vi "jsq_encode.vi"(8 "error in (no error)":errorcluster, 10 "Sequence":T1[](array[typedef])) -> (0 "error out":errorcluster, 2 "JSON string":string="[\r\n]")   [LabVIEW 2015, in "oskar_tools.lvlib"]
uses:
  oskar_tools.lvlib
  seq_line.ctl
  <vilib>/regexp/Match Regular Expression.xnode
  <vilib>/addons/_JKI.lib/Serialization/JSON/JKI JSON Serialization.lvlib
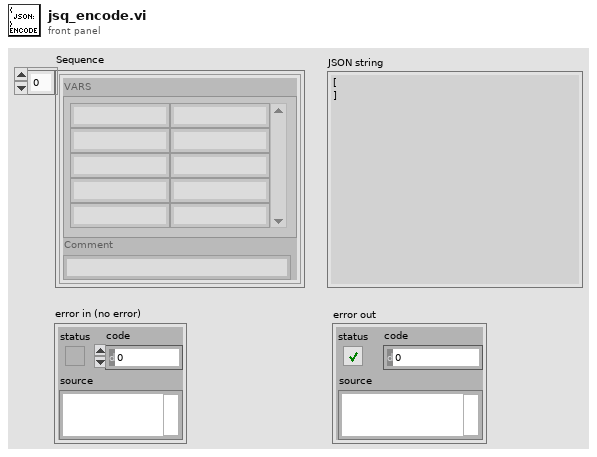
[diagram p1: front panel]
types:
  T1 = typedef "oskar_tools.lvlib/seq_line.ctl" = cluster{"VARS":string[][], "Comment":string}
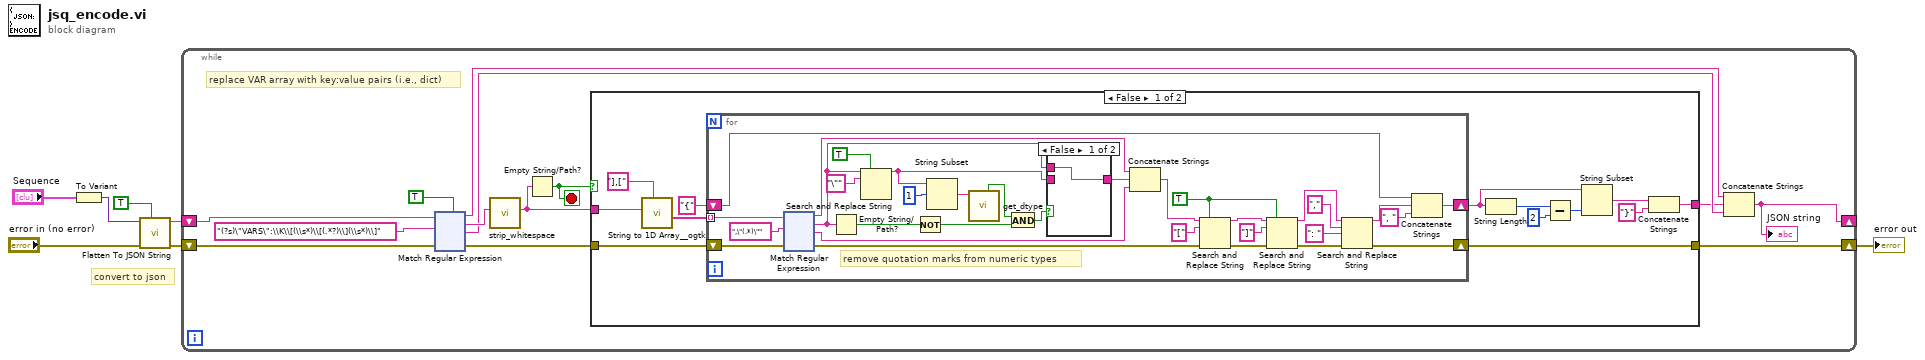
[diagram p0: block diagram]
diagram:
  # "convert to json"
  n1 = To Variant(anything="Sequence") -> (Variant=w7:variant)
  n2 = call <vilib>:"Flatten To JSON String.vi"("Multiline (T)"=TRUE, "error in (no error)"="error in (no error)", "Variant"=w7) -> ("error out"=w2:errorcluster, "JSON String"=w4:string)  [unwired: 7 in]
  n3 = while {
    shift-right: [w17] -> _
    shift-left: w4 -> [w19]
    shift-right: [w8] -> w1
    shift-left: w2 -> [w10]
    stop <- w15 stop-if-true
    # "replace VAR array with key:value pairs (i.e., dict)"
    n4 = xnode "Match Regular Expression"("input string"=w19, "regular expression"="(?s)\"VARS\":\\K\\[(\\s*)\\[(.*?)\\](\\s*)\\]", "error in"=w10, "multiline? (F)"=TRUE) -> ("before match"=w18:string, "whole match"=w14:string, "after match"=w12:string, "error out"=w9:errorcluster)  [unwired: 2 in, 1 out]
    n5 = call "strip_whitespace.vi"("String in"=w14) -> ("String out"=w13:string)  [unwired: 10 in]
    n6 = Empty String/Path?(string/path=w13) -> (empty?=w15:bool)
    n7 = case shown="False" w15 {
      tunnel: w13 -> [w33 w183]
      tunnel: [w28 w183] -> w11
      tunnel: w9 -> [w22 w182]
      tunnel: [w21 w182] -> w8
      frame False {
        n8 = call <userlib>:"String to 1D Array__ogtk.vi"("delimiter (Tab)"="],[" ("format string"), "string"=w33) -> ("Array of Strings"=w31:string[])  [unwired: 9 in]
        n9 = for {
          tunnel: w31 -> [w53] mode=indexing
          shift-right: [w55] -> w27
          shift-left: "{" ("string") -> [w58]
          shift-right: [w34] -> w21
          shift-left: w22 -> [w38]
          w62 = TRUE ("replace all? (F)")
          # "remove quotation marks from numeric types"
          n10 = xnode "Match Regular Expression"("input string"=w53, "regular expression"=",\"(.*)\"", "error in"=w38) -> ("before match"=w52:string, "whole match"=w45:string, "after match"=w50:string, "error out"=w37:errorcluster)  [unwired: 3 in, 1 out]
          n11 = Empty String/Path?(string/path=w45) -> (empty?=w48:bool)
          n12 = Search and Replace String(replace all?=TRUE ("replace all? (F)"), input string=w45, search string="\"") -> (result string=w43:string)  [unwired: 5 in, 3 out]
          n13 = Not(x=w48) -> (.not. x?=w39:bool)
          n14 = String Subset(string=w43, offset (0)=1) -> (substring=w42:string)  [unwired: 1 in]
          n15 = call "get_dtype.vi"("String"=w42) -> ("IsNumber"=w40:bool)  [unwired: 5 in, 5 out]
          n16 = And(x=w40, y=w39) -> (x .and. y?=w47:bool)
          n17 = case shown="False" w47 {
            tunnel: w45 -> [w66 _]
            tunnel: [w66 w67] -> w51
            tunnel: w43 -> [_ w67]
            frame False {
            }
            frame True {
            }
          }
          n18 = Concatenate Strings(w52, w51, w50) -> (w49:string)
          n19 = Search and Replace String(replace all?=w62, input string=w49, search string="[", error in=w37) -> (result string=w63:string, error out=w36:errorcluster)  [unwired: 4 in, 2 out]
          n20 = Search and Replace String(replace all?=w62, input string=w63, search string="]", error in=w36) -> (result string=w61:string, error out=w35:errorcluster)  [unwired: 4 in, 2 out]
          n21 = Search and Replace String(input string=w61, search string=",", replace string=": " ("replace string (\"\")"), error in=w35) -> (result string=w57:string, error out=w34:errorcluster)  [unwired: 4 in, 2 out]
          n22 = Concatenate Strings(w58, w57, ", " ("string")) -> (w55:string)
        }
        n23 = String Length(string=w27) -> (length=w25:i32)
        n24 = Subtract(x=w25, y=2) -> (x-y=w23:i32)
        n25 = String Subset(string=w27, length (rest)=w23) -> (substring=w26:string)  [unwired: 1 in]
        n26 = Concatenate Strings(w26, "}" ("string")) -> (w28:string)
      }
      frame True {
      }
    }
    n27 = Concatenate Strings(w18, w11, w12) -> (w17:string)
    "JSON string" <- w17
  }
  "error out" <- w1
